vi "Untitled 1.vi"() -> ()   [LabVIEW 2024]
uses:
  State.ctl
panel:
  in  "?":T1
  in  "?":T1
  in  "Enum":T1
  in  "?":bool
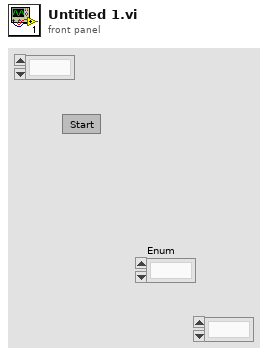
[diagram p1: front panel]
types:
  T1 = typedef "State.ctl" = enum16{""}
  T2 = typedef "State.ctl" = enum16{"Standby", "Stop", "Start"}
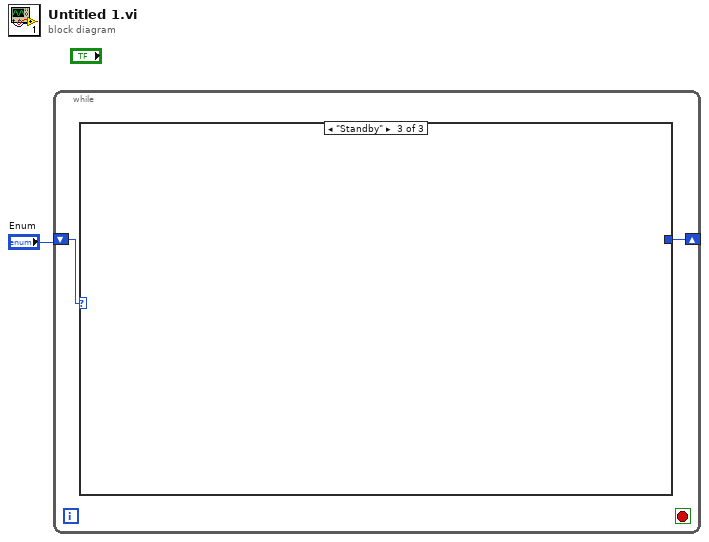
[diagram p0: block diagram]
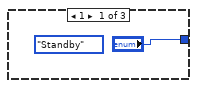
[diagram p2: hidden frame]
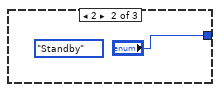
[diagram p3: hidden frame]
diagram:
  n1 = while {
    shift-right: [w3] -> _
    shift-left: "Enum" -> [w2]
    stop <- _ stop-if-true
    n2 = case shown="\"Standby\"" w2 {
      tunnel: ["?" "?" _] -> w3
      frame 1 {
        (unwired) State."Standby"
      }
      frame 2 {
        (unwired) State."Standby"
      }
      frame "" {
      }
    }
  }
